vi "Join byte.vi"(1 "lo":fxp<+,4,4> format="%04b", 2 "hi":fxp<+,4,4> format="%04b") -> (0 "hi.lo":u8 format="%08b")   [LabVIEW 2016]
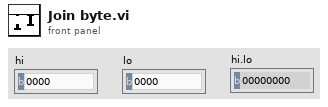
[diagram p1: front panel]
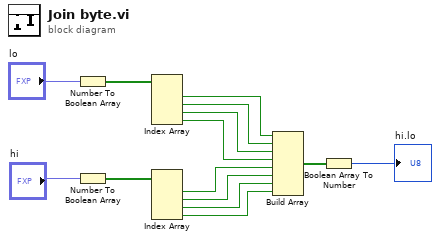
[diagram p0: block diagram]
diagram:
  n1 = Number To Boolean Array(number="lo") -> (Boolean array=w14:bool[])
  n2 = Number To Boolean Array(number="hi") -> (Boolean array=w13:bool[])
  n3 = Index Array(array=w14) -> (element #1=w12:bool, element #2=w11:bool, element #3=w10:bool, element #4=w9:bool)  [unwired: 4 in]
  n4 = Index Array(array=w13) -> (element #1=w8:bool, element #2=w7:bool, element #3=w6:bool, element #4=w5:bool)  [unwired: 4 in]
  n5 = Build Array(w12, w11, w10, w9, w8, w7, w6, w5) -> (w4:bool[])
  n6 = Boolean Array To Number(Boolean array=w4) -> (number=→"hi.lo":u8)
